vi "testAttributeQuotesDouble.vi"(8 "error in (no error)":errorcluster, 11 "TestCase in":refnum<class "EasyXMLTest.lvclass">) -> (0 "error out":errorcluster, 3 "TestCase out":refnum<class "EasyXMLTest.lvclass">)   [LabVIEW 2011, in "EasyXMLTest.lvclass"]
doc: "Verify that error in is not overwritten"
uses:
  EasyXMLTest.lvclass
panel:
  out "Produced Data":variant
  out "Input Data":variant
  out "XML String":string
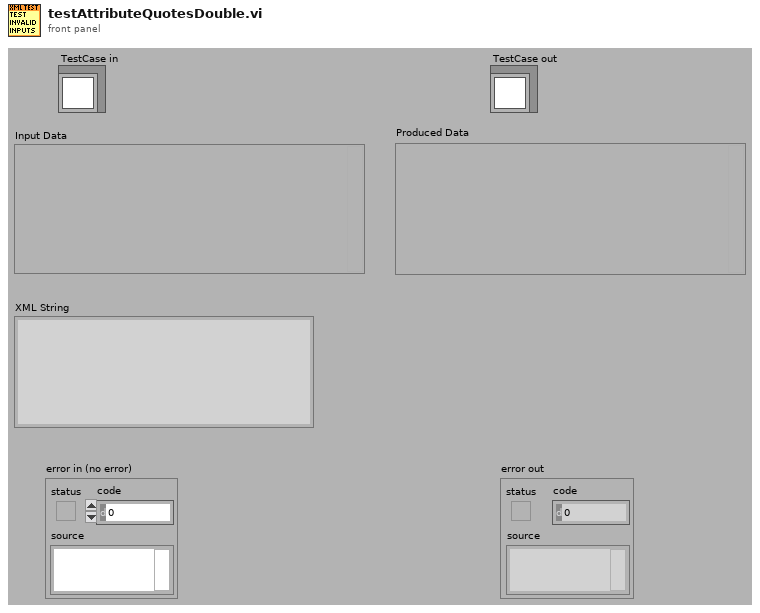
[diagram p1: front panel]
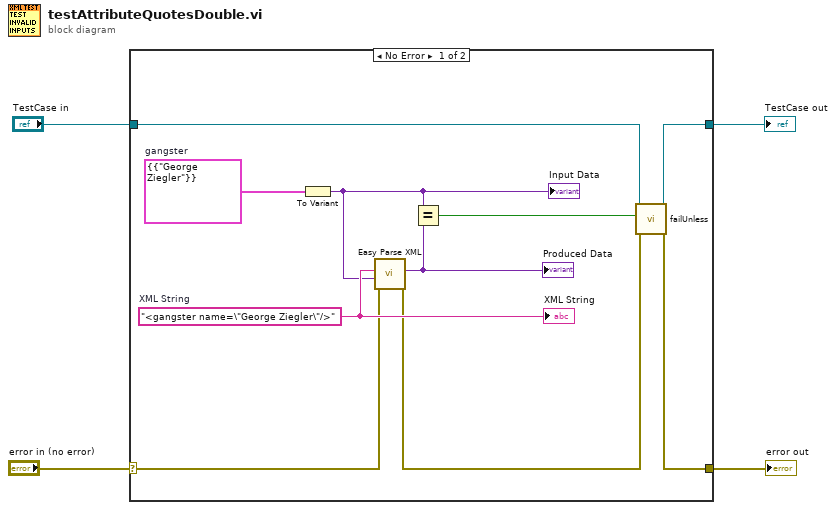
[diagram p0: block diagram]
diagram:
  n1 = case shown="No Error" "error in (no error)" {
    selector: "error in (no error)" -> [w6 w16]
    tunnel: [w9 w16] -> w2
    tunnel: [w7 w15] -> w1
    tunnel: "TestCase in" -> [w8 w15]
    frame No Error {
      w14 = cluster{"#attributes":cluster{"name":string}} {"#attributes"={"name"="George Ziegler"}}  # gangster
      w13 = "<gangster name=\"George Ziegler\"/>"  # XML String
      n2 = To Variant(anything=w14) -> (Variant=w12:variant)
      "Input Data" <- w12
      n3 = call "Easy Parse XML.vi"("error in (no error)"=w6, "LabVIEW Data (Type)"=w12, "XML String"=w13) -> ("error out"=w5:errorcluster, "LabVIEW Data"=w11:variant)  [unwired: 7 in]
      "Produced Data" <- w11
      n4 = Equal?(x=w12, y=w11) -> (x = y?=w10:bool)
      n5 = call-dynamic "failUnless.vi"("error in (no error)"=w5, "pass"=w10, "TestCase in"=w8) -> ("error out"=w9:errorcluster, "TestCase out"=w7:refnum<class "EasyXMLTest.lvclass">)  [unwired: 7 in]
      "XML String" <- w13
    }
    frame Error {
    }
  }
  "error out" <- w2
  "TestCase out" <- w1
